vi "initialize resistance params.vi"(8 "error in (no error)":errorcluster, 9 "hw channel info":T4[](array[typedef]), 10 "instrument handle in":T7, 11 "Data Access Engine in":refnum<class "Data Access Engine.lvclass">) -> (0 "error out":errorcluster, 2 "resistance params":T1, 3 "Data Access Engine out":refnum<class "Data Access Engine.lvclass">)   [LabVIEW 2017, in "NI 272x Resistive Simulation Custom Device Engine.lvlib"]
uses:
  NI 272x Resistive Simulation Custom Device Engine.lvlib
  <instrlib>/ni272xReferenceVIs/ni272xReferenceVIs.llb/ni272x Reference.ctl
  Controls/Compiled HW Channel.ctl
  Controls/Channel Mode.ctl
  <instrlib>/ni272xReferenceVIs/ni272xReferenceVIs.llb/ni272x Callendar-Van Dusen RTD Parameters.ctl
  <vilib>/NI/NIVS Inline Async API/_Data Access Engine/Data Access Engine/Data Access Engine.lvclass
  resistance params.ctl
  <vilib>/NI/NIVS Inline Async API/_Data Access Engine/Data Access Engine/Types/Write.DVR.ctl
  <vilib>/NI/NIVS Inline Async API/_Data Access Engine/Access Type Classes/Write/Write.lvclass
  <vilib>/NI/NIVS Inline Async API/_Data Access Engine/Data Access Engine/Types/Read.DVR.ctl
  <vilib>/NI/NIVS Inline Async API/_Data Access Engine/Access Type Classes/Read/Read.lvclass
  <vilib>/NI/NIVS Inline Async API/_Data Access Engine/Access Type Classes/Write/Write.lvclass/Write.ctl
  <vilib>/NI/NIVS Inline Async API/_Data Access Engine/Data Access Engine/Methods/Write.Data.vi
  <vilib>/NI/NIVS Inline Async API/_Data Access Engine/Access Type Classes/Write/Write.ProcessData.vi
  Globals/Names.vi
  <vilib>/NI/NIVS Inline Async API/_Data Access Engine/Data Access Engine/Methods/Write.Lookup.vi
  <vilib>/NI/NIVS Inline Async API/_Data Access Engine/Data Access Engine/Methods/Read.Lookup.vi
  NI 272x Resistive Simulation Custom Device Shared.lvlib
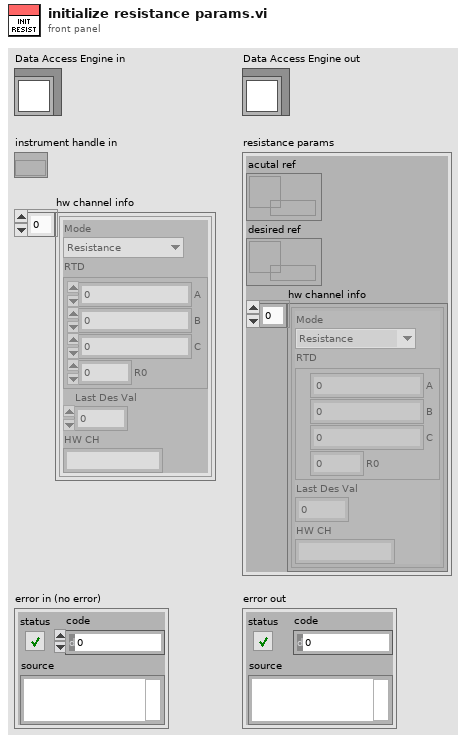
[diagram p1: front panel]
types:
  T1 = typedef "NI 272x Resistive Simulation Custom Device Engine.lvlib/resistance params.ctl" = cluster{"acutal ref":T2, "desired ref":T3, "hw channel info":T4[]}
  T2 = typedef "Data Access Engine.lvlib/Data Access Engine.lvclass/Write.DVR.ctl" = refnum<data-value>
  T3 = typedef "Data Access Engine.lvlib/Data Access Engine.lvclass/Read.DVR.ctl" = refnum<data-value>
  T4 = typedef "NI 272x Resistive Simulation Custom Device Shared.lvlib/Compiled HW Channel.ctl" = cluster{"Mode":T5, "RTD":T6, "Last Des Val":dbl, "HW CH":string}
  T5 = typedef "NI 272x Resistive Simulation Custom Device Shared.lvlib/Channel Mode.ctl" = enum16{"Resistance", "RTD Temperature"}
  T6 = typedef "ni272x Callendar-Van Dusen RTD Parameters.ctl" = cluster{"A":dbl, "B":dbl, "C":dbl, "R0":dbl}
  T7 = typedef "ni272x Reference.ctl" = refnum<k20>
  T8 = cluster{"acutal ref":T2, "desired ref":T3, "hw channel info":T4[]}
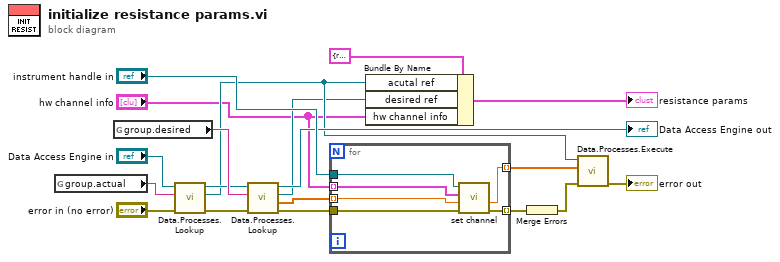
[diagram p0: block diagram]
diagram:
  n1 = global read "Names.vi" "group.actual"() -> (w12:string)
  n2 = global read "Names.vi" "group.desired"() -> (w13:string)
  n3 = call-poly <vilib>:"Data.Processes.Lookup.vi"("error in (no error)"="error in (no error)", "Name"=w12, "Data Access API in"="Data Access Engine in") -> ("error out"=w7:errorcluster, "Ref"=w6:T2, "Data Access API out"=w8:refnum<class "Data Access Engine.lvclass">)  [unwired: 5 in, 1 out]
  n4 = call-poly <vilib>:"Data.Processes.Lookup.vi"("error in (no error)"=w7, "Name"=w13, "Data Access API in"=w8) -> ("error out"=w19:errorcluster, "Initial Values"=w15:dbl[], "Ref"=w5:T3, "Data Access API out"=→"Data Access Engine out":refnum<class "Data Access Engine.lvclass">)  [unwired: 5 in]
  n5 = for {
    tunnel: "hw channel info" -> [w25] mode=indexing
    tunnel: "instrument handle in" -> [w24]
    tunnel: w15 -> [w23] mode=indexing
    tunnel: [w22] -> w16 mode=indexing
    tunnel: [w21] -> w17 mode=indexing
    tunnel: w19 -> [w20]
    n6 = call "set channel.vi"("error in (no error)"=w20, "Channel Data Reference"=w23, "HW Chn"=w25, "Refnum in"=w24) -> ("error out"=w21:errorcluster, "coerced resistance (ohms)"=w22:dbl)  [unwired: 6 in]
  }
  n7 = Bundle By Name(cluster=T8 {"acutal ref"=refnum, "desired ref"=refnum, "hw channel info"=[]}, "acutal ref"=w6, "desired ref"=w5, "hw channel info"="hw channel info") -> (→"resistance params":T8)
  n8 = Merge Errors(w17) -> (w18:errorcluster)
  n9 = call-poly <vilib>:"Data.Processes.Execute.vi"("error in (no error)"=w18, "Values"=w16, "Ref"=w6) -> ("error out"=→"error out":errorcluster)  [unwired: 8 in]
